vi "SCPI Write.vi"(7 "Input String":string, 8 "error in (no error)":errorcluster, 11 "VISA resource name":refnum<visa-resource-name>) -> (0 "error out":errorcluster, 3 "VISA resource name out":refnum<visa-resource-name>)   [LabVIEW 2021, in "BK Precision 169XB.lvlib"]
uses:
  BK Precision 169XB.lvlib
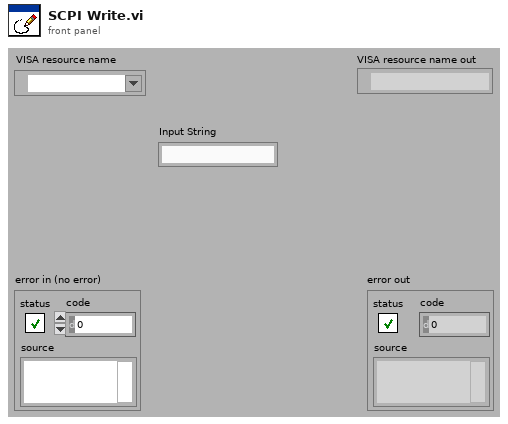
[diagram p1: front panel]
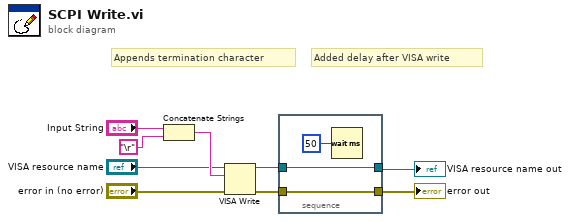
[diagram p0: block diagram]
diagram:
  # "Appends termination character"
  # "Added delay after VISA write"
  n1 = Concatenate Strings("Input String", "\r" ("Carriage Return Constant")) -> (w7:string)
  n2 = VISA Write(VISA resource name="VISA resource name", write buffer=w7, error in (no error)="error in (no error)") -> (VISA resource name out=w6:refnum<visa-resource-name>, error out=w8:errorcluster)  [unwired: 1 out]
  n3 = stacked-sequence {
    tunnel: [w12] -> w2
    tunnel: w8 -> [w12]
    tunnel: w6 -> [w10]
    tunnel: [w10] -> w1
    frame #0 {
      n4 = Wait (ms)(milliseconds to wait=u32 50) -> ()  [unwired: 1 out]
    }
  }
  "error out" <- w2
  "VISA resource name out" <- w1
